vi "FTW-Endpoint-TCP-Multipart-Ask.vi"(0 "FTW Endpoint":refnum<class "FTW-Endpoint-TCP.lvclass">, 5 "Message":T1, 7 "Read Timeout":i32=1000 format="%dmsec", 9 "Write Timeout":i32=-1 format="%dmsec", 11 "error in":errorcluster) -> (4 "FTW Endpoint out":refnum<class "FTW-Endpoint-TCP.lvclass">, 6 "Reply":T1, 8 "Read Timed out?":bool, 10 "Write Timed out?":bool, 15 "error out":errorcluster)   [LabVIEW 2013, in "FTW-Endpoint-TCP.lvclass"]
uses:
  FTW-Endpoint-TCP.lvclass
  Payload/FTW-MessagePayload.ctl
  Ether/FTW-Ether.lvclass
panel:
  # "Inputs"
  # "Outputs"
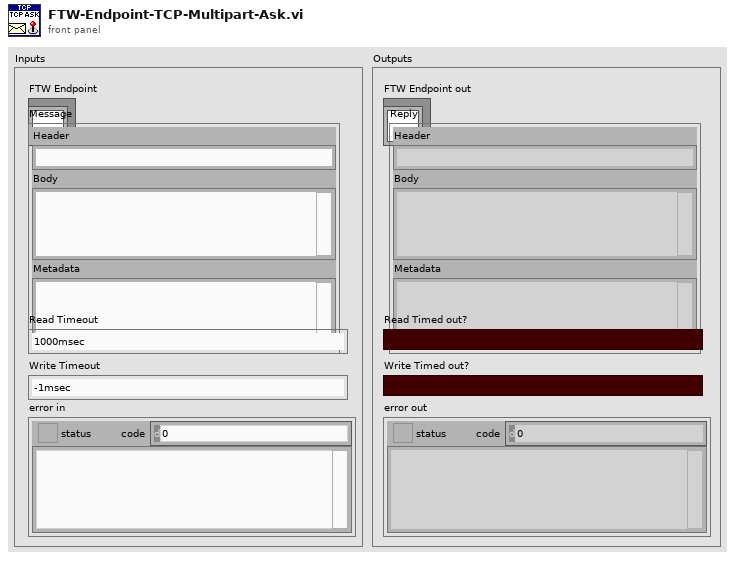
[diagram p1: front panel]
types:
  T1 = typedef "FTW-MessagePayload.ctl" = cluster{"Header":string, "Body":string, "Metadata":string}
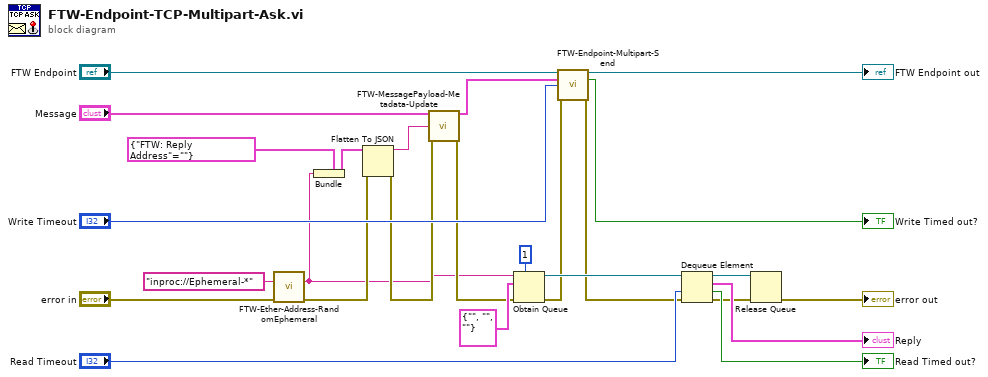
[diagram p0: block diagram]
diagram:
  n1 = call "FTW-Ether-Address-RandomEphemeral.vi"("Endpoint"="inproc://Ephemeral-*" ("Requested Ephemeral Address"), "error in"="error in") -> ("Endpoint with Replacements"=w1:string, "error out"=w4:errorcluster)  [unwired: 12 in]
  n2 = Bundle(cluster=cluster{"FTW: Reply Address":string} {"FTW: Reply Address"=""}, "FTW: Reply Address"=w1) -> (w8:cluster{"FTW: Reply Address":string})
  n3 = Flatten To JSON(anything=w8, error in (no error)=w4) -> (JSON string=w7:string, 11:w3:errorcluster)  [unwired: 1 in]
  n4 = call "FTW-MessagePayload-Metadata-Update.vi"("Message In"="Message", "Metadata"=w7, "error in"=w3) -> ("Message"=w5:T1, "error out"=w2:errorcluster)  [unwired: 11 in]
  n5 = Obtain Queue(max queue size (-1, unlimited)=1, name (unnamed)=w1, element data type=T1 {"Header"="", "Body"="", "Metadata"=""}, error in (no error)=w2) -> (queue out=w12:refnum<queue>, error out=w11:errorcluster)  [unwired: 1 in, 1 out]
  n6 = call-dynamic "FTW-Endpoint-Multipart-Send.vi"("FTW Endpoint"="FTW Endpoint", "Message"=w5, "Timeout"="Write Timeout", "error in"=w11) -> ("FTW Endpoint out"=→"FTW Endpoint out":refnum<class "FTW-Endpoint-TCP.lvclass">, "Timed out?"=→"Write Timed out?":bool, "error out"=w10:errorcluster)  [unwired: 9 in]
  n7 = Dequeue Element(queue=w12, timeout in ms (-1)="Read Timeout", error in (no error)=w10) -> (queue out=w17:refnum<queue>, element=→"Reply":T1, timed out?=→"Read Timed out?":bool, error out=w16:errorcluster)
  n8 = Release Queue(queue=w17, error in (no error)=w16) -> (error out=→"error out":errorcluster)  [unwired: 1 in, 2 out]
